vi "WM Pierson Moskowitz.vi"(0 "Wind Speed":dbl=2.0 caption="m/s (Full Scale)" min=0.0 format="%.2f", 1 "Start Freq (Model Scale)":dbl min=0.0 format="%.2f", 2 "End Freq (Model Scale)":dbl=100.0 min=0.0 format="%.2f", 3 "Scale Ratio":dbl=1.0 min=0.1 format="%.2f", 4 "Number of Frequencies":i32=100 min=2) -> (5 "Spectral Energy":dbl[](array[numeric]) format="%.2f", 6 "PM parameters":cluster{"Wind Speed":dbl, "Scale Ratio":dbl} {"Scale Ratio" format="%.2f"; "Wind Speed" format="%.2f"}, 7 "Frequency":dbl[](array[numeric]) caption="Hz" format="%.2f")   [LabVIEW 2012]
panel:
  in  "Boolean":bool
  # "Pierson Moskowitz"
  # ":1"
  # "Full Scale : Model Scale"
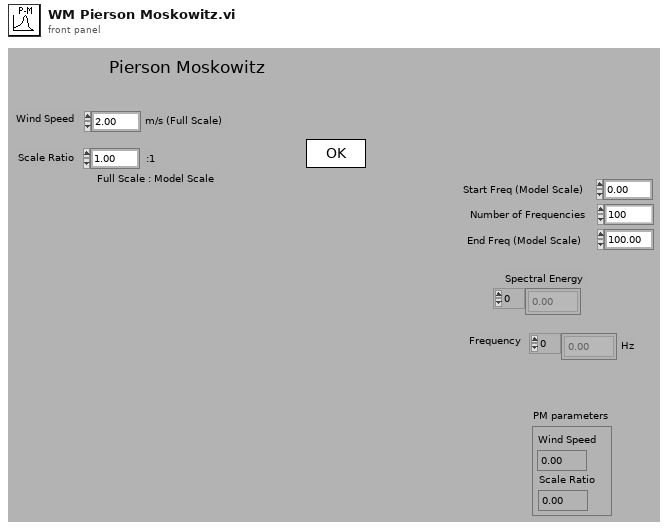
[diagram p1: front panel]
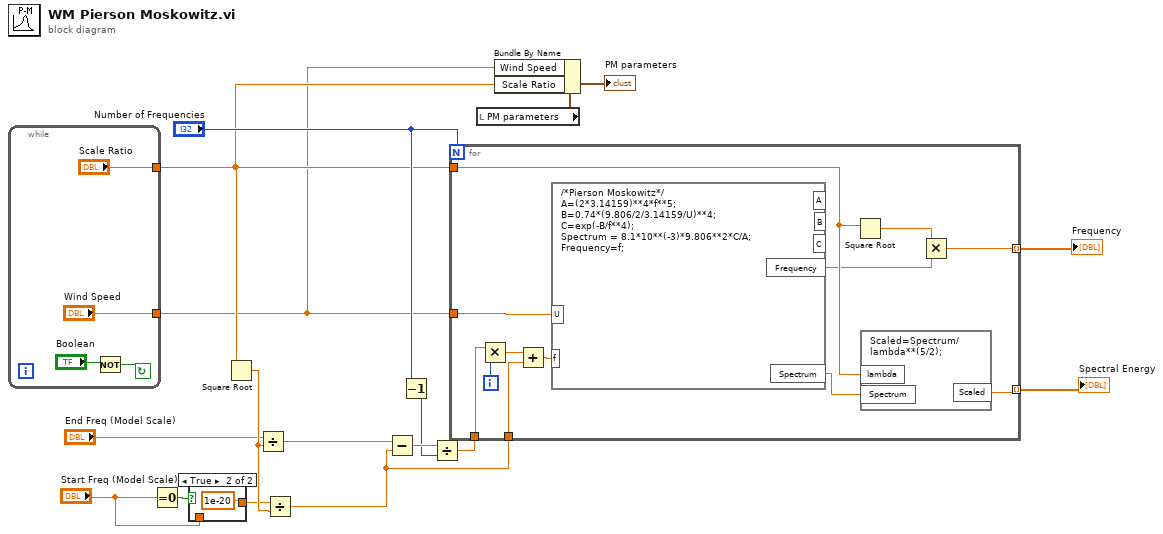
[diagram p0: block diagram]
diagram:
  n1 = while {
    tunnel: ["Wind Speed"] -> w4
    tunnel: ["Scale Ratio"] -> w5
    stop <- w18 continue-if-true
    n2 = Not(x="Boolean") -> (.not. x?=w18:bool)
  }
  n3 = Equal To 0?(x="Start Freq (Model Scale)") -> (x = 0?=w10:bool)
  n4 = case shown="True" w10 {
    tunnel: [w22 1e-20] -> w9
    tunnel: "Start Freq (Model Scale)" -> [w22 _]
    frame False {
    }
    frame True {
    }
  }
  n5 = Square Root(x=w5) -> (sqrt(x)=w13:dbl)
  n6 = Divide(x="End Freq (Model Scale)", y=w13) -> (x/y=w12:dbl)
  n7 = Divide(x=w9, y=w13) -> (x/y=w11:dbl)
  n8 = Subtract(x=w12, y=w11) -> (x-y=w17:dbl)
  n9 = Decrement(x="Number of Frequencies") -> (x-1=w14:i32)
  n10 = Divide(x=w17, y=w14) -> (x/y=w16:dbl)
  n11 = for {
    N: "Number of Frequencies" -> [_]
    tunnel: w4 -> [w35]
    tunnel: [w30] -> w1 mode=indexing
    tunnel: [w27] -> w2 mode=indexing
    tunnel: w11 -> [w31]
    tunnel: w16 -> [w24]
    tunnel: w5 -> [w29]
    i -> [w34]
    n12 = Multiply(x=w24, y=w34) -> (x*y=w32:dbl)
    n13 = Add(x=w32, y=w31) -> (x+y=w33:dbl)
    n14 = formula code="/*Pierson Moskowitz*/\nA=(2*3.14159)**4*f**5;\nB=0.74*(9.806/2/3.14159/U)**4;\nC=exp(-B/f**4);\nSpectrum = 8.1*10**(-3)*9.806**2*C/A;\nFrequency=f;"("U"=w35, "f"=w33) -> ("Spectrum"=w28:dbl, "Frequency"=w25:dbl)  [unwired: 3 out]
    n15 = Square Root(x=w29) -> (sqrt(x)=w26:dbl)
    n16 = formula code="Scaled=Spectrum/lambda**(5/2);"("lambda"=w29, "Spectrum"=w28) -> ("Scaled"=w27:dbl)
    n17 = Multiply(x=w26, y=w25) -> (x*y=w30:dbl)
  }
  "Spectral Energy" <- w2
  "Frequency" <- w1
  n18 = local read "PM parameters"() -> (w6:cluster{"Wind Speed":dbl, "Scale Ratio":dbl})
  n19 = Bundle By Name(cluster=w6, "Wind Speed"=w4, "Scale Ratio"=w5) -> (→"PM parameters":cluster{"Wind Speed":dbl, "Scale Ratio":dbl})
